vi "SwitchLogic.vi"(7 "Deadtime":u8, 9 "enable":bool=TRUE, 10 "triangle":fxp<+/-,32,4>, 11 "sine waves":T1) -> (3 "switch values":bool[](array[boolean]))   [LabVIEW 2015, in "SPWM.lvlib"]
uses:
  SPWM.lvlib
  Signal.ctl
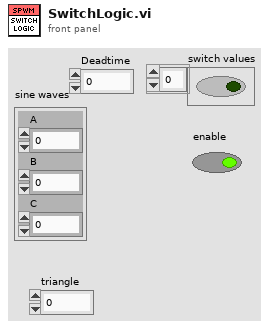
[diagram p1: front panel]
types:
  T1 = typedef "SPWM.lvlib/Signal.ctl" = cluster{"A":fxp<+/-,32,4>, "B":fxp<+/-,32,4>, "C":fxp<+/-,32,4>}
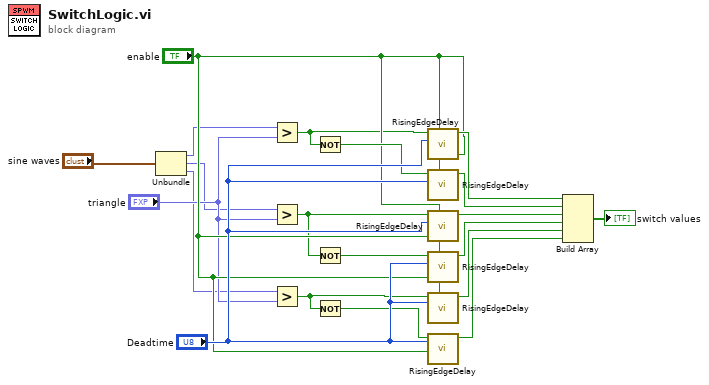
[diagram p0: block diagram]
diagram:
  n1 = Unbundle("sine waves") -> ("A"=w4:fxp<+/-,32,4>, "B"=w2:fxp<+/-,32,4>, "C"=w1:fxp<+/-,32,4>)
  n2 = Greater?(x=w4, y="triangle") -> (0:w8:bool)
  n3 = Greater?(x=w2, y="triangle") -> (0:w7:bool)
  n4 = Greater?(x=w1, y="triangle") -> (0:w6:bool)
  n5 = Not(x=w8) -> (.not. x?=w14:bool)
  n6 = Not(x=w7) -> (.not. x?=w13:bool)
  n7 = Not(x=w6) -> (.not. x?=w12:bool)
  n8 = call "RisingEdgeDelay.vi"("enable?"="enable", "Deadtime (iterations)"="Deadtime", "Input"=w8) -> ("Output"=w19:bool)  [unwired: 8 in]
  n9 = call "RisingEdgeDelay.vi"("enable?"="enable", "Deadtime (iterations)"="Deadtime", "Input"=w14) -> ("Output"=w18:bool)  [unwired: 8 in]
  n10 = call "RisingEdgeDelay.vi"("enable?"="enable", "Deadtime (iterations)"="Deadtime", "Input"=w7) -> ("Output"=w17:bool)  [unwired: 8 in]
  n11 = call "RisingEdgeDelay.vi"("enable?"="enable", "Deadtime (iterations)"="Deadtime", "Input"=w13) -> ("Output"=w16:bool)  [unwired: 8 in]
  n12 = call "RisingEdgeDelay.vi"("enable?"="enable", "Deadtime (iterations)"="Deadtime", "Input"=w6) -> ("Output"=w11:bool)  [unwired: 8 in]
  n13 = call "RisingEdgeDelay.vi"("enable?"="enable", "Deadtime (iterations)"="Deadtime", "Input"=w12) -> ("Output"=w15:bool)  [unwired: 8 in]
  n14 = Build Array(w19, w18, w17, w16, w11, w15) -> (→"switch values":bool[])
